vi "Test Connection.vi"() -> ()   [LabVIEW 2025]
uses:
  <vilib>/LabVIEW Open Source Project/MQTT Control Packets/Control Packets/CONNECT/ConnectFlags -- cluster.ctl
  <vilib>/LabVIEW Open Source Project/MQTT Client/Client class/Client.lvclass/Client.ctl
  <vilib>/LabVIEW Open Source Project/MQTT Connection/MQTT_Base/Base Class/MQTT_Base.lvclass/MQTT_Base.ctl
  <vilib>/LabVIEW Open Source Project/MQTT Control Packets/Control Packets/ControlPacket/ControlPacket.lvclass/ControlPacket.ctl
  <vilib>/LabVIEW Open Source Project/Connection/Connection.TCP/Connection.TCP.lvclass
  C:/Program Files/National Instruments/LabVIEW 2025/vi.lib/LabVIEW Open Source Project/Connection/Connection/Connection.lvclass
  <vilib>/LabVIEW Open Source Project/MQTT Client/Client class/Client.lvclass
  C:/Program Files/National Instruments/LabVIEW 2025/vi.lib/LabVIEW Open Source Project/MQTT Connection/MQTT_Base/Base Class/MQTT_Base.lvclass
  <vilib>/LabVIEW Open Source Project/MQTT Control Packets/Control Packets/PUBLISH/PUBLISH.lvclass
  C:/Program Files/National Instruments/LabVIEW 2025/vi.lib/LabVIEW Open Source Project/MQTT Control Packets/Control Packets/ControlPacket/ControlPacket.lvclass
  <vilib>/LabVIEW Open Source Project/MQTT Connection/MQTT_Base/Base Class/MQTT_Base.lvclass
  <vilib>/LabVIEW Open Source Project/MQTT Control Packets/Control Packets/ControlPacket/ControlPacket.lvclass
  <vilib>/LabVIEW Open Source Project/Connection/Connection.LocalQueue/Connection.LocalQueue.lvclass
  <vilib>/LabVIEW Open Source Project/Connection/Connection/Connection.lvclass
  C:/Program Files/National Instruments/LabVIEW 2025/vi.lib/LabVIEW Open Source Project/MQTT Client/Client class/Client.lvclass
  <vilib>/LabVIEW Open Source Project/MQTT Control Packets/Control Packets/CONNECT/CONNECT.lvclass
  C:/Program Files/National Instruments/LabVIEW 2025/vi.lib/LabVIEW Open Source Project/MQTT Control Packets/Control Packets/PUBLISH/PUBLISH.lvclass
panel:
  out "Incoming Message":u8[](array[numeric]) format="%08b"
  in  "Subscribe":bool
  out "Suback":bool
  out "Published":bool
  in  "Publish":bool
  in  "Stop Client":bool
  out "error out":errorcluster
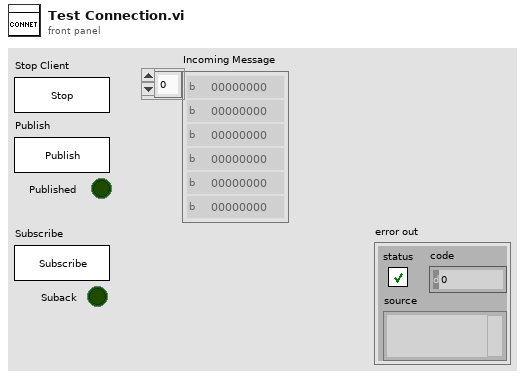
[diagram p1: front panel]
types:
  T1 = typedef "MQTT_Control_Packets.lvlib/CONNECT.lvclass/ConnectFlags -- cluster.ctl" = cluster{"Reserved":bool, "Clean Session":bool, "Will Flag":bool, "Will QoS 1":bool, "Will QoS 2":bool, "Will Retain":bool, "Password Flag":bool, "User Name Flag":bool}
  T2 = cluster{"Will Topic":string, "Will Message":string, "Username":string, "Password":string}
  T3 = typedef "MQTT Client.lvlib/Client.lvclass/Public Events -- cluster.ctl" = cluster{"Connection Status":refnum<user-event>, "Connected":refnum<user-event>, "Application Message":refnum<user-event>}
  T4 = typedef "MQTT Base.lvlib/MQTT_Base.lvclass/Public Events -- cluster.ctl" = cluster{"Stop Event":refnum<user-event>, "Error Event":refnum<user-event>, "Inbound Message":refnum<user-event>}
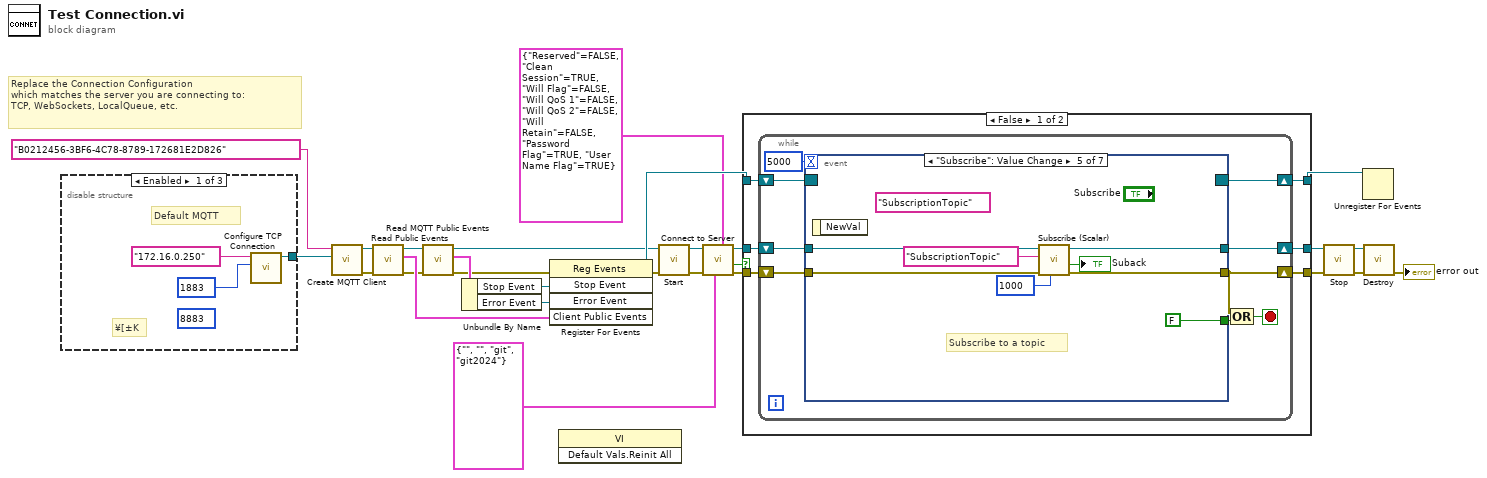
[diagram p0: block diagram]
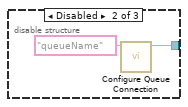
[diagram p2: hidden frame]
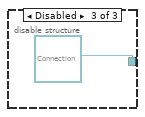
[diagram p3: hidden frame]
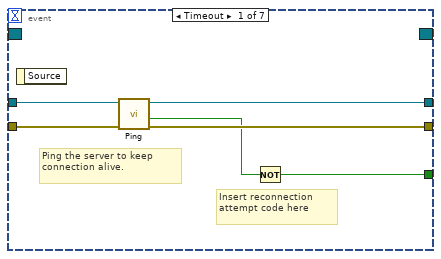
[diagram p4: hidden frame]
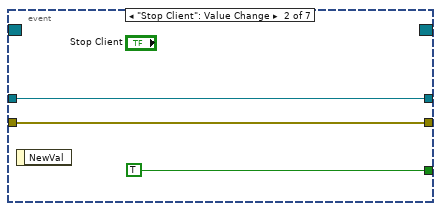
[diagram p5: hidden frame]
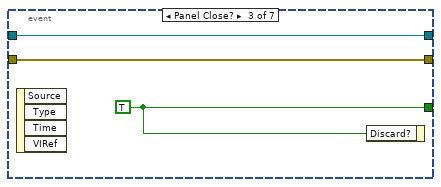
[diagram p6: hidden frame]
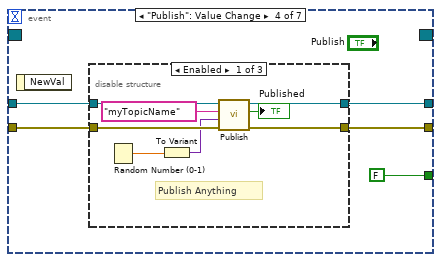
[diagram p7: hidden frame]
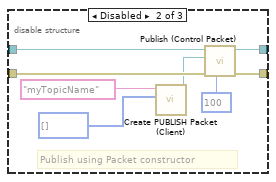
[diagram p8: hidden frame]
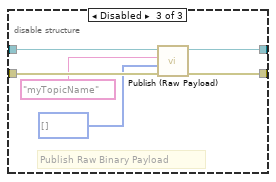
[diagram p9: hidden frame]
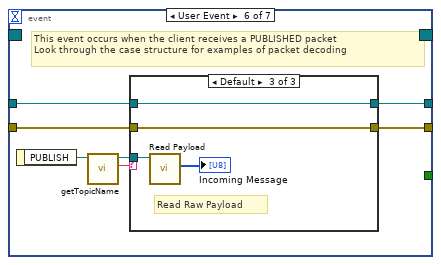
[diagram p10: hidden frame]
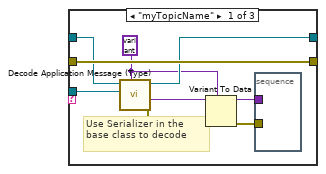
[diagram p11: hidden frame]
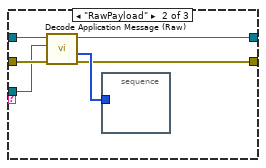
[diagram p12: hidden frame]
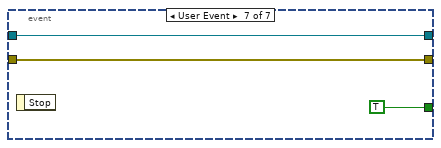
[diagram p13: hidden frame]
diagram:
  # "Replace the Connection Configuration\nwhich matches the server you are connecting to:\nTCP, WebSockets, LocalQueue, etc."
  n1 = disable-structure shown="Enabled" {
    disable-tunnel: [w29 w32 refnum<class "Connection.lvclass"> refnum ("Connection Configuration")] -> w27
    frame Enabled {
      (unwired) u16 8883 ("remote port (80)")
      # "¥[±K"
      # "Default MQTT"
      n2 = call <vilib>:"Configure TCP Connection.vi"("remote port (80)"=u16 1883, "address (localhost)"="172.16.0.250") -> ("Connection.TCP"=w29:refnum<class "Connection.TCP.lvclass">)  [unwired: 8 in, 1 out]
    }
    frame Disabled {
      n3 = call <vilib>:"Configure Queue Connection.vi"("Queue Name"="queueName") -> ("Connection.LocalQueue"=w32:refnum<class "Connection.LocalQueue.lvclass">)  [unwired: 9 in, 1 out]
    }
    frame Disabled {
    }
  }
  n4 = call <vilib>:"Create MQTT Client.vi"("Connection Configuration"=w27, "ID (empty:generate new)"="B0212456-3BF6-4C78-8789-172681E2D826" ("Client ID")) -> ("error out"=w6:errorcluster, "Client out"=w4:refnum<class "Client.lvclass">)  [unwired: 8 in]
  n5 = call <vilib>:"Read Public Events.vi"("error in (no error)"=w6, "Client in"=w4) -> ("error out"=w7:errorcluster, "Client Public Events"=w9:T3, "Client out"=w5:refnum<class "Client.lvclass">)  [unwired: 7 in]
  n6 = call <vilib>:"Read MQTT Public Events.vi"("error in (no error)"=w7, "MQTT_Base in"=w5) -> ("error out"=w8:errorcluster, "MQTT Public Events"=w21:T4, "MQTT_Base out"=w11:refnum<class "Client.lvclass">)  [unwired: 7 in]
  n7 = Unbundle By Name(w21) -> ("Stop Event"=w19:refnum<user-event>, "Error Event"=w20:refnum<user-event>)
  n8 = register-events(error in=w8, w19, w20, w9) -> (reference out=w14:refnum<event-registration>, error out=w10:errorcluster)  [unwired: 1 in]
  n9 = invoke class="VI" method="Default Vals.Reinit All"() -> ()  [unwired: 3 in, 3 out]
  n10 = call <vilib>:"Start.vi"("error in (no error)"=w10, "MQTT_Base in"=w11) -> ("error out"=w13:errorcluster, "MQTT_Base out"=w12:refnum<class "Client.lvclass">)  [unwired: 7 in, 1 out]
  n11 = call <vilib>:"Connect to Server.vi"("Connect Flags"=T1 {"Reserved"=FALSE, "Clean Session"=TRUE, "Will Flag"=FALSE, "Will QoS 1"=FALSE, "Will QoS 2"=FALSE, "Will Retain"=FALSE, "Password Flag"=TRUE, "User Name Flag"=TRUE}, "Payload"=T2 {"Will Topic"="", "Will Message"="", "Username"="git", "Password"="git2024"}, "error in (no error)"=w13, "Client in"=w12) -> ("error out"=w17:errorcluster, "timed out"=w16:bool, "Client out"=w18:refnum<class "Client.lvclass">)  [unwired: 4 in, 1 out]
  n12 = case shown="False" w16 {
    tunnel: w14 -> [w39 w127]
    tunnel: [w38 w127] -> w15
    tunnel: w17 -> [w35 w125]
    tunnel: w18 -> [w37 w126]
    tunnel: [w36 w126] -> w23
    tunnel: [w34 w125] -> w25
    frame False {
      n13 = while {
        shift-right: [w47] -> w38
        shift-left: w39 -> [w48]
        shift-right: [w40] -> w36
        shift-left: w37 -> [w41]
        shift-right: [w45] -> w34
        shift-left: w35 -> [w46]
        stop <- w44 stop-if-true
        n14 = event shown="[4] \"Subscribe\": Value Change" {
          selector: w48 -> [_ _ _ _ _ _ _]
          dyn-events: [_ _ _ _ _ _ _] -> w47
          timeout: 5000 -> [_ _ _ _ _ _ _]
          tunnel: w46 -> [w53 w56 w58 w63 w92 w97 w124]
          tunnel: [w51 w56 w58 w62 w91 w98 w124] -> w45
          tunnel: [w50 TRUE w60 FALSE FALSE _ TRUE] -> w43
          tunnel: w41 -> [w54 w57 w59 w64 w94 w100 w122]
          tunnel: [w52 w57 w59 w61 w90 w99 w122] -> w40
          event Timeout {
            # "Insert reconnection\nattempt code here"
            # "Ping the server to keep\nconnection alive."
            n15 = event-data() -> ()  [unwired: 1 in, 1 out]
            n16 = call <vilib>:"Ping.vi"("error in (no error)"=w53, "Client in"=w54) -> ("error out"=w51:errorcluster, "Server responded"=w49:bool, "Client out"=w52:refnum<class "Client.lvclass">)  [unwired: 6 in, 1 out]
            n17 = Not(x=w49) -> (.not. x?=w50:bool)
          }
          event "Stop Client": Value Change {
            n18 = event-data() -> ()  [unwired: 1 in, 1 out]
          }
          event Panel Close? {
            w60 = TRUE
            n19 = event-data() -> ()  [unwired: 1 in, 4 out]
            n20 = event-data("Discard?"=w60) -> ()  [unwired: 1 in, 1 out]
          }
          event "Publish": Value Change {
            n21 = event-data() -> ()  [unwired: 1 in, 1 out]
            n22 = disable-structure shown="Enabled" {
              disable-tunnel: w64 -> [w73 w79 w87]
              disable-tunnel: w63 -> [w72 w77 w84]
              disable-tunnel: [w71 w76 w85] -> w62
              disable-tunnel: [w70 w78 w86] -> w61
              frame Enabled {
                # "Publish Anything"
                n23 = Random Number (0-1)() -> (number: 0 to 1=w68:dbl)
                n24 = To Variant(anything=w68) -> (Variant=w67:variant)
                n25 = call <vilib>:"Publish.vi"("error in (no error)"=w72, "Payload"=w67, "Topic Name (empty: Payload name)"="myTopicName", "Client in"=w73) -> ("error out"=w71:errorcluster, "Published"=→"Published":bool, "Client out"=w70:refnum<class "Client.lvclass">)  [unwired: 5 in]
              }
              frame Disabled {
                # "Publish using Packet constructor"
                n26 = call <vilib>:"Create PUBLISH Packet (Client).vi"("Payload"=u8[] [], "Topic Name"="myTopicName" ("Topic Name (empty: Payload name)")) -> ("PUBLISH"=w74:refnum<class "PUBLISH.lvclass">)  [unwired: 6 in, 3 out]
                n27 = call <vilib>:"Publish (Control Packet).vi"("timeout (1000ms)"=100 ("timeout (0ms : no ack)"), "error in (no error)"=w77, "PUBLISH"=w74, "Client in"=w79) -> ("error out"=w76:errorcluster, "Client out"=w78:refnum<class "Client.lvclass">)  [unwired: 5 in, 1 out]
              }
              frame Disabled {
                # "Publish Raw Binary Payload"
                n28 = call <vilib>:"Publish (Raw Payload).vi"("error in (no error)"=w84, "Binary Payload"=u8[] [] ("Payload"), "Topic Name"="myTopicName" ("Topic Name (empty: Payload name)"), "Client in"=w87) -> ("error out"=w85:errorcluster, "Client out"=w86:refnum<class "Client.lvclass">)  [unwired: 5 in, 1 out]
              }
            }
          }
          event "Subscribe": Value Change {
            (unwired) "SubscriptionTopic" ("Topic Name (empty: Payload name)")
            # "Subscribe to a topic"
            n29 = event-data() -> ()  [unwired: 1 in, 1 out]
            n30 = call <vilib>:"Subscribe (Scalar).vi"("timeout (1000ms)"=1000 ("timeout (100ms)"), "error in (no error)"=w92, "Topic Filter"="SubscriptionTopic" ("Topic Name (empty: Payload name)"), "Client in"=w94) -> ("error out"=w91:errorcluster, "Ack"=→"Suback":bool, "Client out"=w90:refnum<class "Client.lvclass">)  [unwired: 5 in]
          }
          event User Event {
            # "This event occurs when the client receives a PUBLISHED packet\nLook through the case structure for examples of packet decoding"
            n31 = event-data() -> ("PUBLISH"=w102:refnum<class "PUBLISH.lvclass">)  [unwired: 1 in]
            n32 = call <vilib>:"getTopicName.vi"("PUBLISH in"=w102) -> ("Topic"=w101:string, "PUBLISH out"=w96:refnum<class "PUBLISH.lvclass">)  [unwired: 8 in, 1 out]
            n33 = case shown="Default" w101 {
              tunnel: w100 -> [w108 w117 w121]
              tunnel: [w107 w116 w121] -> w99
              tunnel: [w111 w114 w120] -> w98
              tunnel: w97 -> [w111 w113 w120]
              tunnel: w96 -> [w106 w112 w119]
              frame "myTopicName" {
                w104 = variant ("Type")
                # "Use Serializer in the\nbase class to decode"
                n34 = call <vilib>:"Decode Application Message (Type).vi"("Type"=w104, "PUBLISH"=w106, "Client in"=w108) -> ("error out"=w103:errorcluster, "Payload"=w105:variant, "Client out"=w107:refnum<class "Client.lvclass">)  [unwired: 5 in, 1 out]
                n35 = Variant To Data(error in=w103, type=w104, Variant=w105) -> (data=w110:variant, error out=w109:errorcluster)
                n36 = stacked-sequence {
                  tunnel: w110 -> [_]
                  tunnel: w109 -> [_]
                  frame #0 {
                  }
                }
              }
              frame "RawPayload" {
                n37 = call <vilib>:"Decode Application Message (Raw).vi"("error in (no error)"=w113, "PUBLISH"=w112, "Client in"=w117) -> ("error out"=w114:errorcluster, "Payload"=w115:u8[], "Client out"=w116:refnum<class "Client.lvclass">)  [unwired: 5 in, 1 out]
                n38 = stacked-sequence {
                  tunnel: w115 -> [_]
                  frame #0 {
                  }
                }
              }
              frame Default {
                # "Read Raw Payload"
                n39 = call <vilib>:"Read Payload.vi"("ControlPacket in"=w119) -> ("Payload"=→"Incoming Message":u8[])  [unwired: 9 in, 1 out]
              }
            }
          }
          event User Event {
            n40 = event-data() -> ()  [unwired: 1 in, 1 out]
          }
        }
        n41 = Compound Arithmetic op=OR(w45, w43) -> (w44:bool)
      }
    }
    frame True {
    }
  }
  n42 = call <vilib>:"Stop.vi"("error in (no error)"=w25, "MQTT_Base in"=w23) -> ("error out"=w24:errorcluster, "MQTT_Base out"=w22:refnum<class "Client.lvclass">)  [unwired: 7 in, 1 out]
  n43 = Unregister For Events(event registration refnum=w15) -> ()  [unwired: 1 in, 1 out]
  n44 = call <vilib>:"Destroy.vi"("error in (no error)"=w24, "MQTT_Base in"=w22) -> ("error out"=→"error out":errorcluster)  [unwired: 8 in, 1 out]
